vi "Get Nested Property Name.vi"(10 "property key name":string, 11 "property base name":string) -> (3 "full property name":string)   [LabVIEW 2017, in "Routing and Faulting Scripting.lvlib"]
uses:
  Routing and Faulting Scripting.lvlib
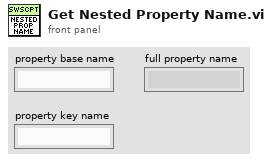
[diagram p1: front panel]
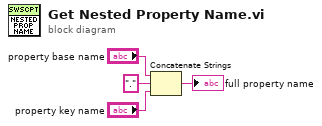
[diagram p0: block diagram]
diagram:
  n1 = Concatenate Strings("property base name", "." ("string"), "property key name") -> (→"full property name":string)
